vi "solar_qtimer Get QTimers.vi"(11 "QTimer Refnum":T1) -> (2 "QTimers":T2[](array[typedef]), 3 "QTimer Names":string[](array[string]), 5 "Valid Refnum?":bool)   [LabVIEW 2018]
doc: "This returns the list of QTimers in the instance reference."
uses:
  solar_qtimer_ctl QTimer.ctl
  solar_qtimer_ctl Refnum.ctl
  solar_qtimer_ctl QTimer Settings.ctl
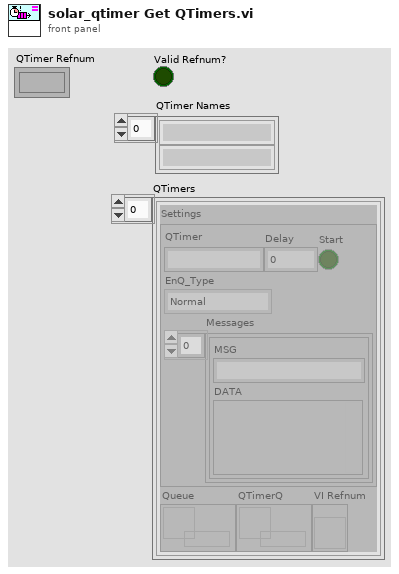
[diagram p1: front panel]
types:
  T1 = typedef "solar_qtimer_ctl Refnum.ctl" = refnum<k1>
  T2 = typedef "solar_qtimer_ctl QTimer.ctl" = cluster{"Settings":T3, "Queue":refnum<queue>, "QTimerQ":refnum<queue>, "VI Refnum":refnum<vi>}
  T3 = typedef "solar_qtimer_ctl QTimer Settings.ctl" = cluster{"QTimer":string, "Delay":i32, "Start":bool, "EnQ_Type":enum8{"Normal", "Priority", "IgnoreIfExists"}, "Messages":cluster{"MSG":string, "DATA":variant}[]}
  T4 = typedef "solar_qtimer_ctl SEQ.ctl" = cluster{"QTimers":T2[]}
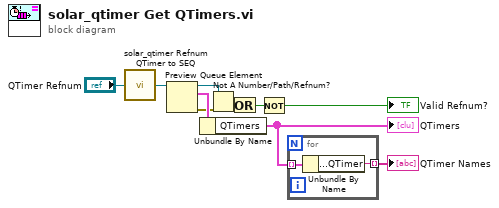
[diagram p0: block diagram]
diagram:
  n1 = call "solar_qtimer Refnum QTimer to SEQ.vi"("QTimer Refnum"="QTimer Refnum") -> ("QTimers SEQ"=w8:refnum<queue>)
  n2 = Preview Queue Element(queue=w8) -> (queue out=w5:refnum<queue>, element=w10:T4, error out=w4:errorcluster)  [unwired: 2 in, 1 out]
  n3 = Unbundle By Name(w10) -> ("QTimers"=w2:T2[])
  "QTimers" <- w2
  n4 = Not A Number/Path/Refnum?(number/path/refnum=w5) -> (NaN/Path/Refnum?=w7:bool)
  n5 = Or(x=w7, y=w4) -> (x .or. y?=w6:bool)
  n6 = Not(x=w6) -> (.not. x?=→"Valid Refnum?":bool)
  n7 = for {
    tunnel: w2 -> [w12] mode=indexing
    tunnel: [w11] -> w1 mode=indexing
    n8 = Unbundle By Name(w12) -> ("Settings.QTimer"=w11:string)
  }
  "QTimer Names" <- w1
